vi "RNN_Backward_Pass_demo_alt2.vi"() -> ()   [LabVIEW 2014]
uses:
  <vilib>/Analysis/Matrix/Datatypes/RealMatrix.ctl
  <vilib>/Analysis/baseanly.llb/A x Vector.vi
  <vilib>/Analysis/Matrix/Numeric/Conversions/Array To Matrix - RA.vi
  <vilib>/Analysis/Matrix/Numeric/Add/Add - RM,RM.vi
  <vilib>/Analysis/Matrix/NI_Matrix.lvlib
  <vilib>/Analysis/NI_AALBase.lvlib
panel:
  in  "_params":T2={"Wxh"=[[0.578129, 2.569937, -0.0219857], [-2.46959, 0.027262, 2.449614362]], "Whh"=[[-1.3996, 0.961745], [0.364566, -0.477064]], "bh"=[[0.535351], [-1.985987]], "Why"=[[-0.658616, 0.764692], [-1.7789986, 0.388036], [-0.130912, -0.333988]], "by"=[[-0.528417], [-0.44032], [-0.8844819]]} {"Wxh" format="%_8f"; "Whh" format="%_8f"; "bh" format="%_8f"; "Why" format="%_8f"; "by" format="%_8f"}
  out "dParams_":T3={"Real Matrix"=[[0.0, 0.00198618922483572, 0.0], [0.0, -0.0611889253874036, 0.0]], "Real Matrix"=[[0.0, 0.0], [0.0, 0.0]], "Real Matrix (Column Vector)"=[[0.00198618922483572], [-0.0611889253874036]], "Real Matrix"=[[-0.79352176628, 0.76563674128], [0.10403833634399999, -0.100382341344], [0.689482433944, -0.665253438944]], "Real Matrix (Column Vector)"=[[-0.7967150000000001], [0.104457], [0.692257]]}
  out "dy":dbl[](array[numeric])=[-0.7967150000000001, 0.104457, 0.692257] format="%_8f"
  out "dhnext (out)":dbl[](array[numeric])=[-0.025087272211864256, 0.031101241057055938] format="%_8f"
  out "dhnext (in)":dbl[](array[numeric]) format="%_8f"
  out "dhraw":dbl[](array[numeric])=[0.00198618922483572, -0.0611889253874036] format="%_8f"
  out "dh":dbl[](array[numeric])=[0.24827564129580007, -0.7999140412440001] format="%_8f"
  out "hs[t]":dbl[](array[numeric])=[0.995992, -0.960992] format="%_8f"
  out "hs[t-1]":dbl[](array[numeric]) format="%_8f"
  in  "t --->  t - 1":bool
  out "t":i32
  out "t (reversed)":i32
  out "input length":i32=1
  out "dby":T1=[[-0.7967150000000001], [0.104457], [0.692257]] format="%_8f"
  out "dbh":T1=[[0.00198618922483572], [-0.0611889253874036]] format="%_8f"
  out "dWhy":T1=[[-0.79352176628, 0.76563674128], [0.10403833634399999, -0.100382341344], [0.689482433944, -0.665253438944]] format="%_8f"
  out "dWhh":T1 format="%_8f"
  out "dWxh":T1=[[0.0, 0.00198618922483572, 0.0], [0.0, -0.0611889253874036, 0.0]] format="%_8f"
  in  "targets":i32[](array[numeric])=[0]
  in  "hs":dbl[][][](array[numeric])=[[[0.0], [0.0]], [[0.995992], [-0.960992]]] format="%_8f"
  in  "ps":dbl[][][](array[numeric])=[[[0.203285], [0.104457], [0.692257]]] format="%_8f"
  in  "xs":dbl[][][](array[numeric])=[[[0.0], [1.0], [0.0]]]
  # "dParams"
  # "temporary variables"
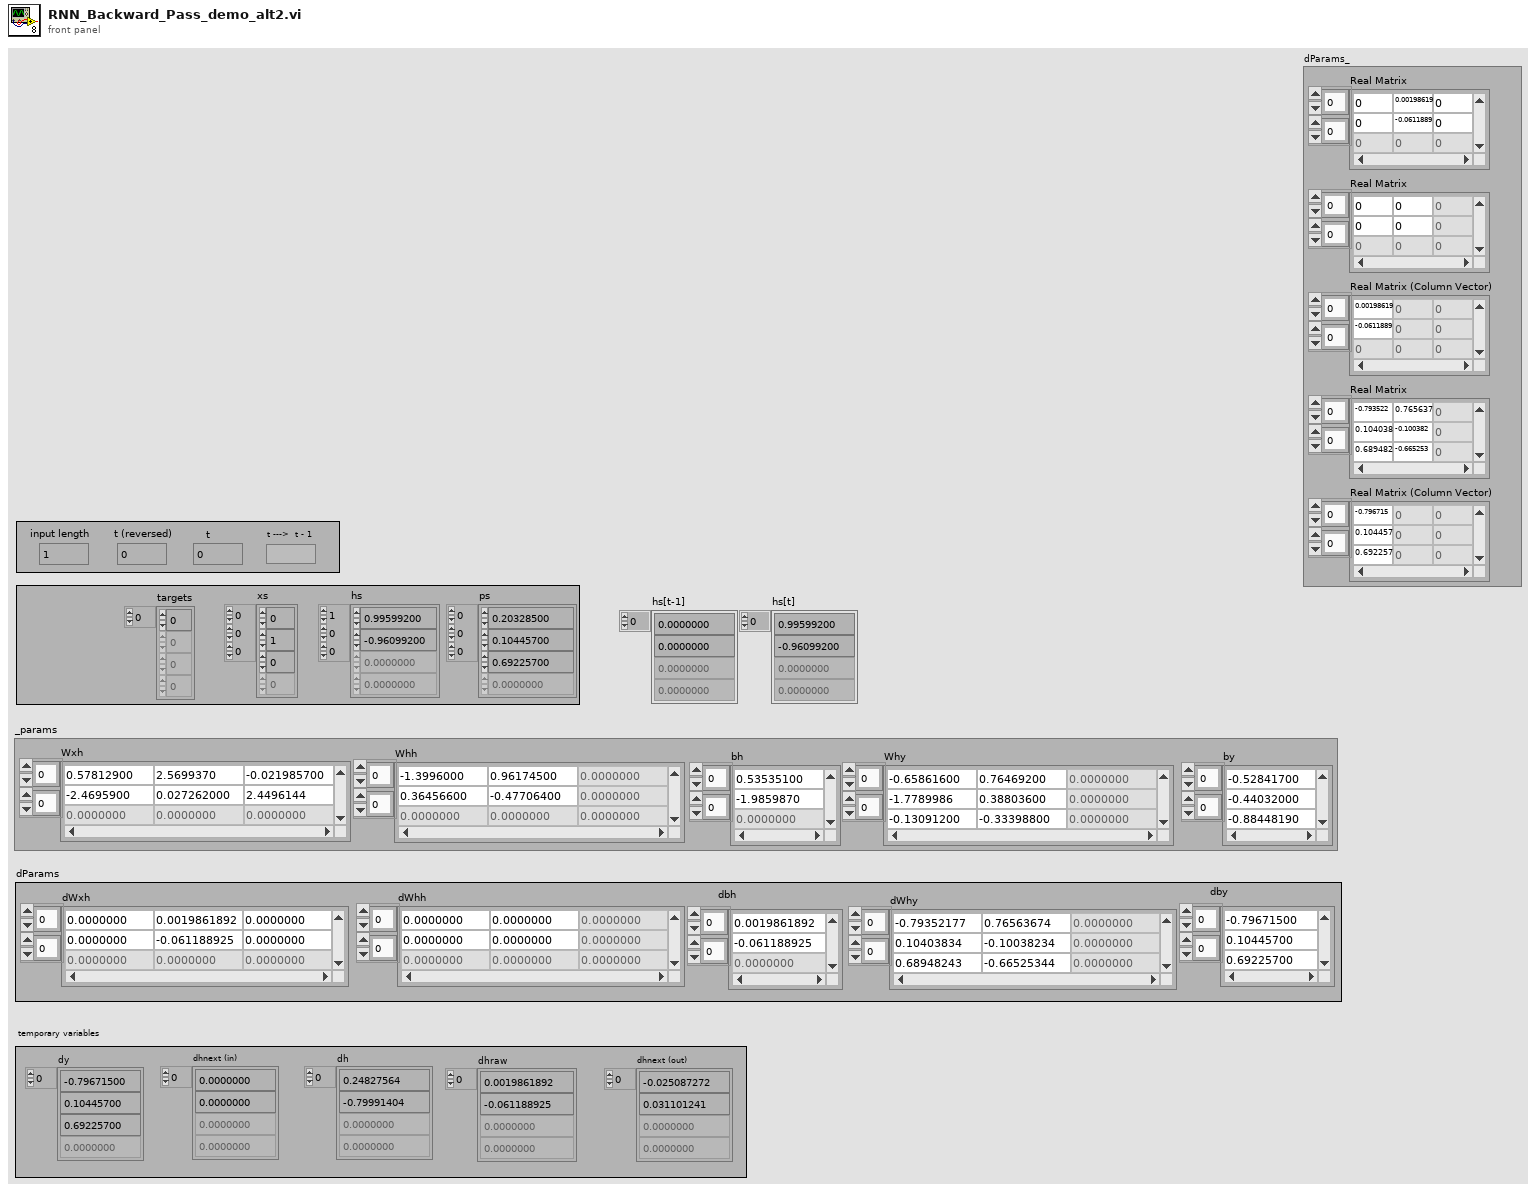
[diagram p1: front panel]
types:
  T1 = typedef "NI_Matrix.lvlib/RealMatrix.ctl" = dbl[][]
  T2 = cluster{"Wxh":T1, "Whh":T1, "bh":T1, "Why":T1, "by":T1}
  T3 = cluster{"Real Matrix":T1, "Real Matrix":T1, "Real Matrix (Column Vector)":T1, "Real Matrix":T1, "Real Matrix (Column Vector)":T1}
  T4 = cluster{"A + B":T1, "A + B":T1, "Real Matrix (Column Vector)":T1, "A + B":T1, "Real Matrix (Column Vector)":T1}
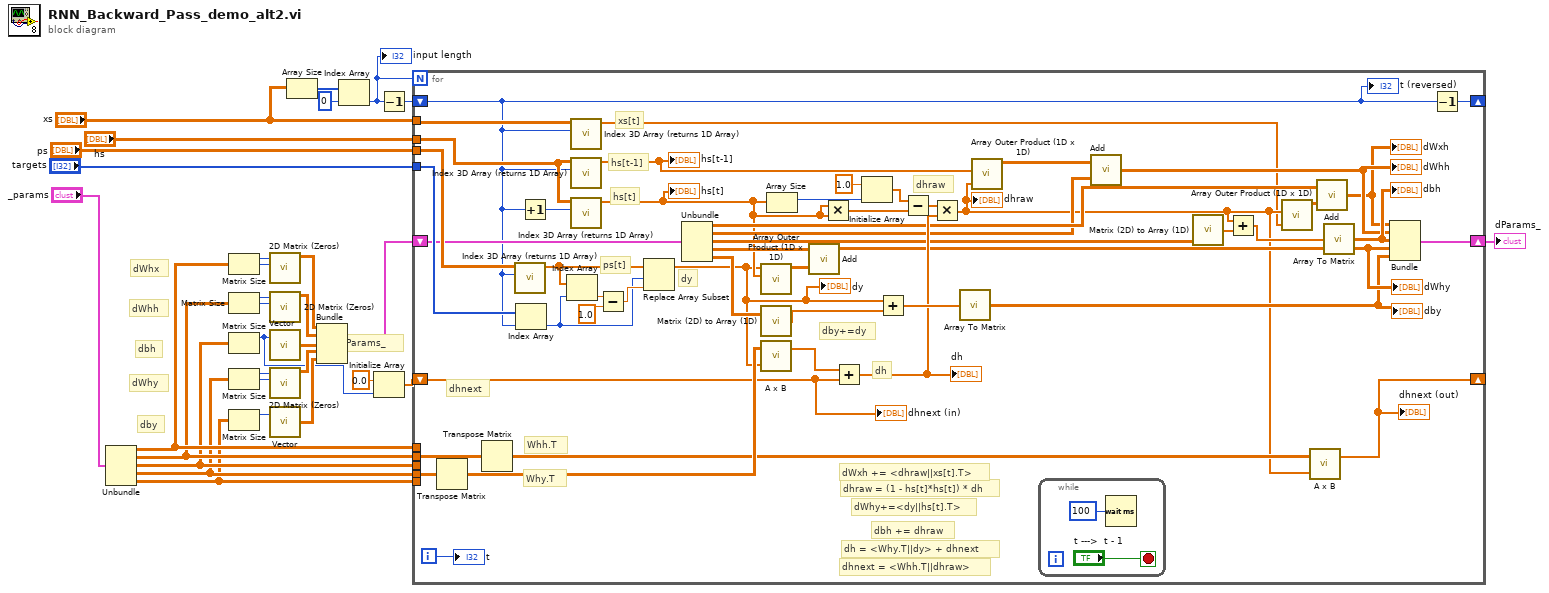
[diagram p0: block diagram]
diagram:
  # "dWhx"
  # "dWhh"
  # "dby"
  # "dWhy"
  # "dbh"
  # "dParams_"
  n1 = Unbundle("_params") -> ("Wxh"=w10:T1, "Whh"=w9:T1, "bh"=w8:T1, "Why"=w7:T1, "by"=w6:T1)
  n2 = Matrix Size(0:w10) -> (1:w12:i32, 2:w21:i32)
  n3 = Matrix Size(0:w9) -> (1:w23:i32, 2:w22:i32)
  n4 = Matrix Size(0:w8) -> (1:w15:i32)  [unwired: 1 out]
  n5 = Matrix Size(0:w7) -> (1:w25:i32, 2:w24:i32)
  n6 = Matrix Size(0:w6) -> (1:w26:i32)  [unwired: 1 out]
  n7 = call "2D Matrix (Zeros).vi"("nCols (1)"=w21, "nRows"=w12) -> ("Real Matrix"=w16:T1)  [unwired: 9 in]
  n8 = call "2D Matrix (Zeros).vi"("nCols (1)"=w22, "nRows"=w23) -> ("Real Matrix"=w17:T1)  [unwired: 9 in]
  n9 = call "Vector.vi"("length"=w15) -> ("Real Matrix (Column Vector)"=w18:T1)  [unwired: 1 in]
  n10 = call "2D Matrix (Zeros).vi"("nCols (1)"=w24, "nRows"=w25) -> ("Real Matrix"=w19:T1)  [unwired: 9 in]
  n11 = call "Vector.vi"("length"=w26) -> ("Real Matrix (Column Vector)"=w20:T1)  [unwired: 1 in]
  n12 = Array Size(array="xs") -> (size(s)=w4:i32[])
  n13 = Bundle("Real Matrix"=w16, "Real Matrix"=w17, "Real Matrix (Column Vector)"=w18, "Real Matrix"=w19, "Real Matrix (Column Vector)"=w20) -> (w28:T3)  [unwired: 1 in]
  n14 = Index Array(array=w4, index=0) -> (element=w2:i32)
  "input length" <- w2
  n15 = Initialize Array(0.0 ("element"), w15) -> (w13:dbl[])
  n16 = Decrement(x=w2) -> (x-1=w27:i32)
  n17 = for {
    N: w2 -> [_]
    shift-right: [w51] -> w11
    shift-left: w28 -> [w69]
    tunnel: "xs" -> [w34]
    tunnel: "hs" -> [w77]
    tunnel: "ps" -> [w78]
    shift-right: [w80] -> _
    shift-left: w27 -> [w32]
    tunnel: "targets" -> [w79]
    shift-right: [w35] -> _
    shift-left: w13 -> [w39]
    tunnel: w7 -> [w50]
    tunnel: w9 -> [w49]
    tunnel: w10 -> [_]
    tunnel: w6 -> [_]
    tunnel: w8 -> [_]
    i -> [w81]
    # "dhnext = <Whh.T||dhraw>"
    # "dWxh += <dhraw||xs[t].T>"
    # "dbh += dhraw"
    # "dhraw = (1 - hs[t]*hs[t]) * dh"
    # "dh = <Why.T||dy> + dhnext"
    # "dWhy+=<dy||hs[t].T>"
    # "xs[t]"
    # "dhnext"
    # "Whh.T"
    # "dy"
    # "dhraw"
    # "dh"
    # "Why.T"
    # "dby+=dy"
    # "hs[t-1]"
    # "hs[t]"
    # "ps[t]"
    n18 = Transpose Matrix(1:w50) -> (0:w65:T1)
    n19 = Transpose Matrix(1:w49) -> (0:w54:T1)
    n20 = call "Index 3D Array (returns 1D Array).vi"("index"=w32, "3D array"=w78) -> ("1D array"=w74:dbl[])  [unwired: 9 in]
    n21 = Index Array(array=w79, index=w32) -> (element=w72:i32)
    n22 = Increment(x=w32) -> (x+1=w48:i32)
    n23 = Index Array(array=w74, index=w72) -> (element=w76:dbl)
    n24 = call "Index 3D Array (returns 1D Array).vi"("index"=w32, "3D array"=w34) -> ("1D array"=w33:dbl[])  [unwired: 9 in]
    n25 = call "Index 3D Array (returns 1D Array).vi"("index"=w32, "3D array"=w77) -> ("1D array"=w53:dbl[])  [unwired: 9 in]
    "hs[t-1]" <- w53
    n26 = call "Index 3D Array (returns 1D Array).vi"("index"=w48, "3D array"=w77) -> ("1D array"=w37:dbl[])  [unwired: 9 in]
    "hs[t]" <- w37
    n27 = Subtract(x=w76, y=1.0) -> (x-y=w73:dbl)
    n28 = Replace Array Subset(array=w74, new element=w73, index=w72) -> (w36:dbl[])
    "dy" <- w36
    n29 = Unbundle(w69) -> ("Real Matrix"=w56:T1, "Real Matrix"=w42:T1, "Real Matrix (Column Vector)"=w57:T1, "Real Matrix"=w67:T1, "Real Matrix (Column Vector)"=w68:T1)
    n30 = call "Array Outer Product (1D x 1D).vi"("array b"=w37, "array a"=w36) -> ("a X b"=w66:dbl[][])  [unwired: 9 in]
    n31 = call "Matrix (2D) to Array (1D).vi"("Matrix (2D)"=w68) -> ("Array (1D)"=w70:dbl[])  [unwired: 4 in]
    n32 = call-poly <vilib>:"A x B.vi"("Vector"=w36, "A"=w65) -> ("A x Vector"=w64:dbl[])  [unwired: 1 out]
    n33 = Array Size(array=w37) -> (size(s)=w63:i32)
    n34 = call-poly <vilib>:"Add.vi"("Real Matrix B"=w66, "Real Matrix A"=w67) -> ("A + B"=w47:T1)
    "dWhy" <- w47
    n35 = Multiply(x=w37, y=w37) -> (x*y=w60:dbl[])
    n36 = Add ("Add.vi")(x=w64, y=w39) -> (x+y=w59:dbl[])
    "dh" <- w59
    n37 = Initialize Array(1.0 ("element"), w63) -> (w61:dbl[])
    n38 = Add(x=w36, y=w70) -> (x+y=w71:dbl[])
    n39 = Subtract(x=w61, y=w60) -> (x-y=w58:dbl[])
    n40 = Multiply(x=w58, y=w59) -> (x*y=w38:dbl[])
    "dhraw" <- w38
    n41 = call-poly <vilib>:"Array To Matrix.vi"("Real 1D Array"=w71) -> ("Real Matrix (Column Vector)"=w46:T1)
    "dby" <- w46
    n42 = call "Array Outer Product (1D x 1D).vi"("array b"=w53, "array a"=w38) -> ("a X b"=w41:dbl[][])  [unwired: 9 in]
    n43 = while {
      stop <- "t --->  t - 1" stop-if-true
      n44 = Wait (ms)(milliseconds to wait=u32 100) -> ()  [unwired: 1 out]
    }
    n45 = call-poly <vilib>:"Add.vi"("Real Matrix B"=w42, "Real Matrix A"=w41) -> ("A + B"=w44:T1)
    "dWhh" <- w44
    n46 = call "Matrix (2D) to Array (1D).vi"("Matrix (2D)"=w57) -> ("Array (1D)"=w40:dbl[])  [unwired: 4 in]
    n47 = Add ("Add.vi")(x=w38, y=w40) -> (x+y=w52:dbl[])
    n48 = call "Array Outer Product (1D x 1D).vi"("array b"=w33, "array a"=w38) -> ("a X b"=w55:dbl[][])  [unwired: 9 in]
    n49 = call-poly <vilib>:"A x B.vi"("Vector"=w38, "A"=w54) -> ("A x Vector"=w35:dbl[])  [unwired: 1 out]
    "dhnext (out)" <- w35
    n50 = call-poly <vilib>:"Add.vi"("Real Matrix B"=w55, "Real Matrix A"=w56) -> ("A + B"=w43:T1)
    "dWxh" <- w43
    n51 = call-poly <vilib>:"Array To Matrix.vi"("Real 1D Array"=w52) -> ("Real Matrix (Column Vector)"=w45:T1)
    "dbh" <- w45
    n52 = Bundle("A + B"=w43, "A + B"=w44, "Real Matrix (Column Vector)"=w45, "A + B"=w47, "Real Matrix (Column Vector)"=w46) -> (w51:T4)  [unwired: 1 in]
    n53 = Decrement(x=w32) -> (x-1=w80:i32)
    "t" <- w81
    "t (reversed)" <- w32
    "dhnext (in)" <- w39
  }
  "dParams_" <- w11
